vi "inverter.vi"(8 "invert":bool, 11 "input":u32 format="%x") -> (0 "output":u32 format="%x")   [LabVIEW 2014]
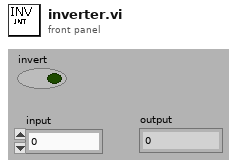
[diagram p1: front panel]
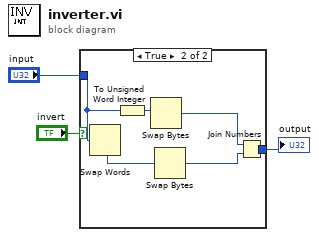
[diagram p0: block diagram]
diagram:
  n1 = case shown="True" "invert" {
    tunnel: "input" -> [w4 w10]
    tunnel: [w4 w5] -> w2
    frame False {
    }
    frame True {
      n2 = Swap Words(1:w10) -> (0:w8:u32)
      n3 = To Unsigned Word Integer(number=w10) -> (unsigned 16bit integer=w9:u16)
      n4 = Swap Bytes(anything=w9) -> (byte swapped=w7:u16)
      n5 = Swap Bytes(anything=w8) -> (byte swapped=w6:u32)
      n6 = Join Numbers(hi=w7, lo=w6) -> ((hi.lo)=w5:u64)
    }
  }
  "output" <- w2
